vi "Main.vi"() -> ()   [LabVIEW 2011]
panel:
  in  "Button_1":bool
  in  "Button_0":bool
  in  "Button_Plus":bool
  in  "Display":string
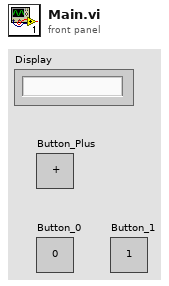
[diagram p1: front panel]
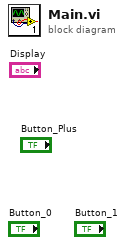
[diagram p0: block diagram]
diagram:
